vi "Main (DAQ, 3 Tasks, Event Messenger).vi"() -> ()   [LabVIEW 2018]
doc: "Datenerfassung - Producer/Consumer mit Zustandsmaschine und Tag Channel\n\n* Analoges Eingangssigna, Definition des\nDAQmx Kanals im NI Max\n* Realisierung mit eine Zustandsmaschine\n* Drei Schleifen (Tasks): Zustandsmaschine und Datenerfassung und Auswertung\n*Realisierung des User Interfaces mit Event Structure\n* Kommunikation benutzereingaben (Zustandsmaschine) zu Datenerfassung mit \"Tag Channel\" und \"Stream Channel\"\n* Anzeige der Events\n* Anzeige der Zustände \"Messung/Warten/Auswertung\""
uses:
  Type Definitions/States UI.ctl
  Type Definitions/MessungEvents.ctl
  <vilib>/DAQmx/read.llb/DAQmx Read (Analog Wfm 1Chan NSamp).vi
  <extravilib>/ChannelInstances/Stream-wfm(dbl)/Read With Abort.vi
  <extravilib>/ChannelInstances/Stream-wfm(dbl)/Write With Abort.vi
  <extravilib>/ChannelInstances/Stream-wfm(dbl)/EndpointRead.vi
  <extravilib>/ChannelInstances/Stream-wfm(dbl)/Endpoint.vi
  <extravilib>/ChannelInstances/Event Messenger-t'MessungEvents.ctl'/Instantiate.vi
  <extravilib>/ChannelInstances/Event Messenger-t'MessungEvents.ctl'/))Channel.vi
  <extravilib>/ChannelInstances/Stream-wfm(dbl)/Instantiate.vi
  <extravilib>/ChannelInstances/Stream-wfm(dbl)/)Channel.vi
  <resource>/ChannelSupport/_ChannelSupport/WaitIfNeeded.vi
  <vilib>/Waveform/WDTOps.llb/WDT Append Waveforms DBL.vi
  <vilib>/DAQmx/miscellaneous.llb/DAQmx Fill In Error Info.vi
  <extravilib>/ChannelInstances/Stream-wfm(dbl).lvlib
  <extravilib>/ChannelInstances/Event Messenger-t'MessungEvents.ctl'.lvlib
panel:
  in  "Tab Control":enum32{"Graph", "Chart"}(tab)=enum."Chart"
  out "element":waveform(dbl)(graph)
  out "Waveform Chart":waveform(dbl)(graph)
  out "Messung":bool
  out "Events":string="Exit= 1"
  in  "Messung":bool
  in  "Exit":bool
  out "Anzeige":dbl(knob) scale=0.0..10.0 scale format="%1.1f"
  # "Datenerfassung - Producer/Consumer mit Zustandsmaschine und Tag sowie Stream Channel\n\n* Analoges Eingangssignal, Definition des\nDAQmx Kanals im NI Max\n*  Realisierung mit eine Zustandsmaschine\n* Zustandsmaschine nur für UI Events\n* Drei Schleifen (Tasks): Zustandsmaschine, Datenerfassung und Auswertung\n*Realisierung des User Interfaces mit Event Structure\n* Kommunikation Benutzereingaben (Zustandsmaschine) zu Datenerfassung mit \"Event Messages\"\n* Daten per Stream Channel zum Zustand \"Auswertung\"\n* Anzeige der Events\n* Anzeige der Zustände \"Messung/Warten/Auswertung\"\n\nTiming\n* Task 1Khz Sampling Rate und 100 Samples\n* Gemessen jede 1sec (Timed loop)\n\nBug\nnur eine Scan!"
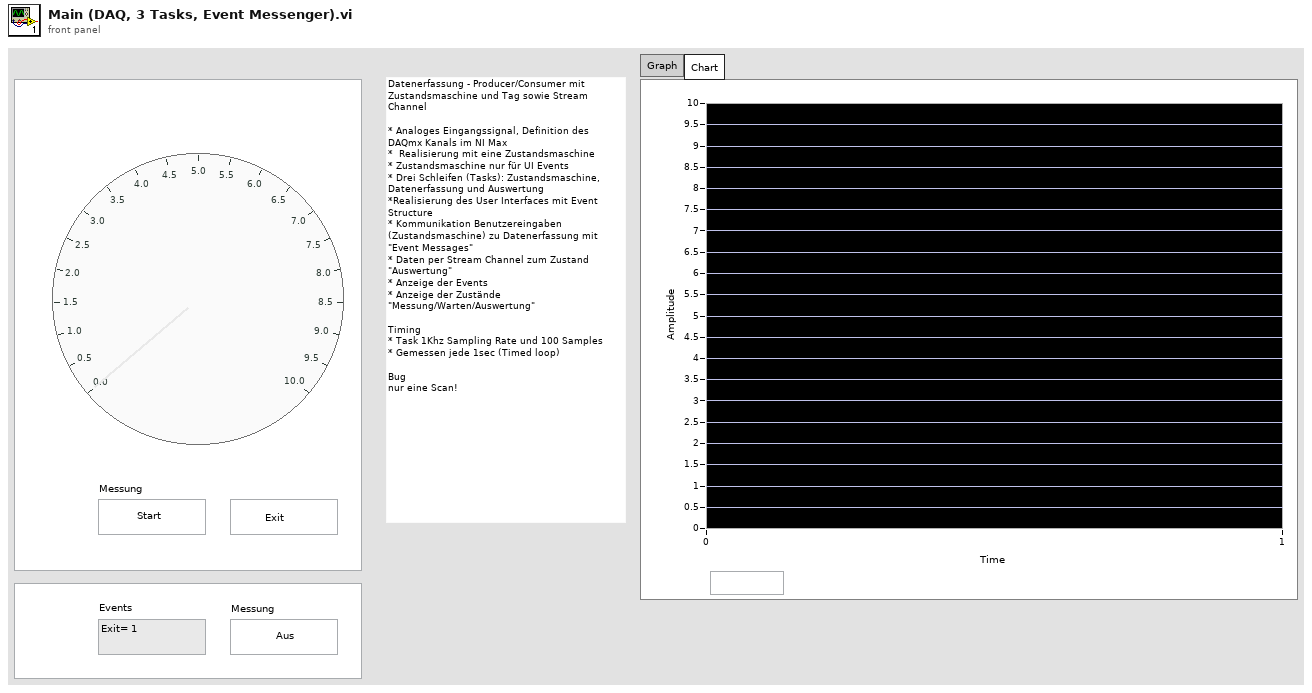
[diagram p1: front panel]
types:
  T1 = typedef "States UI.ctl" = enum16{"Initialize", "Wait for Event", "Exit"}
  T2 = typedef "MessungEvents.ctl" = enum16{"Starten", "Pausieren", "Stoppen"}
  T3 = typedef "Event Messenger-t'MessungEvents.ctl'.lvlib/))Channel.ctl" = refnum<queue>
  T4 = typedef "Stream-wfm(dbl).lvlib/)Channel.ctl" = refnum<queue>
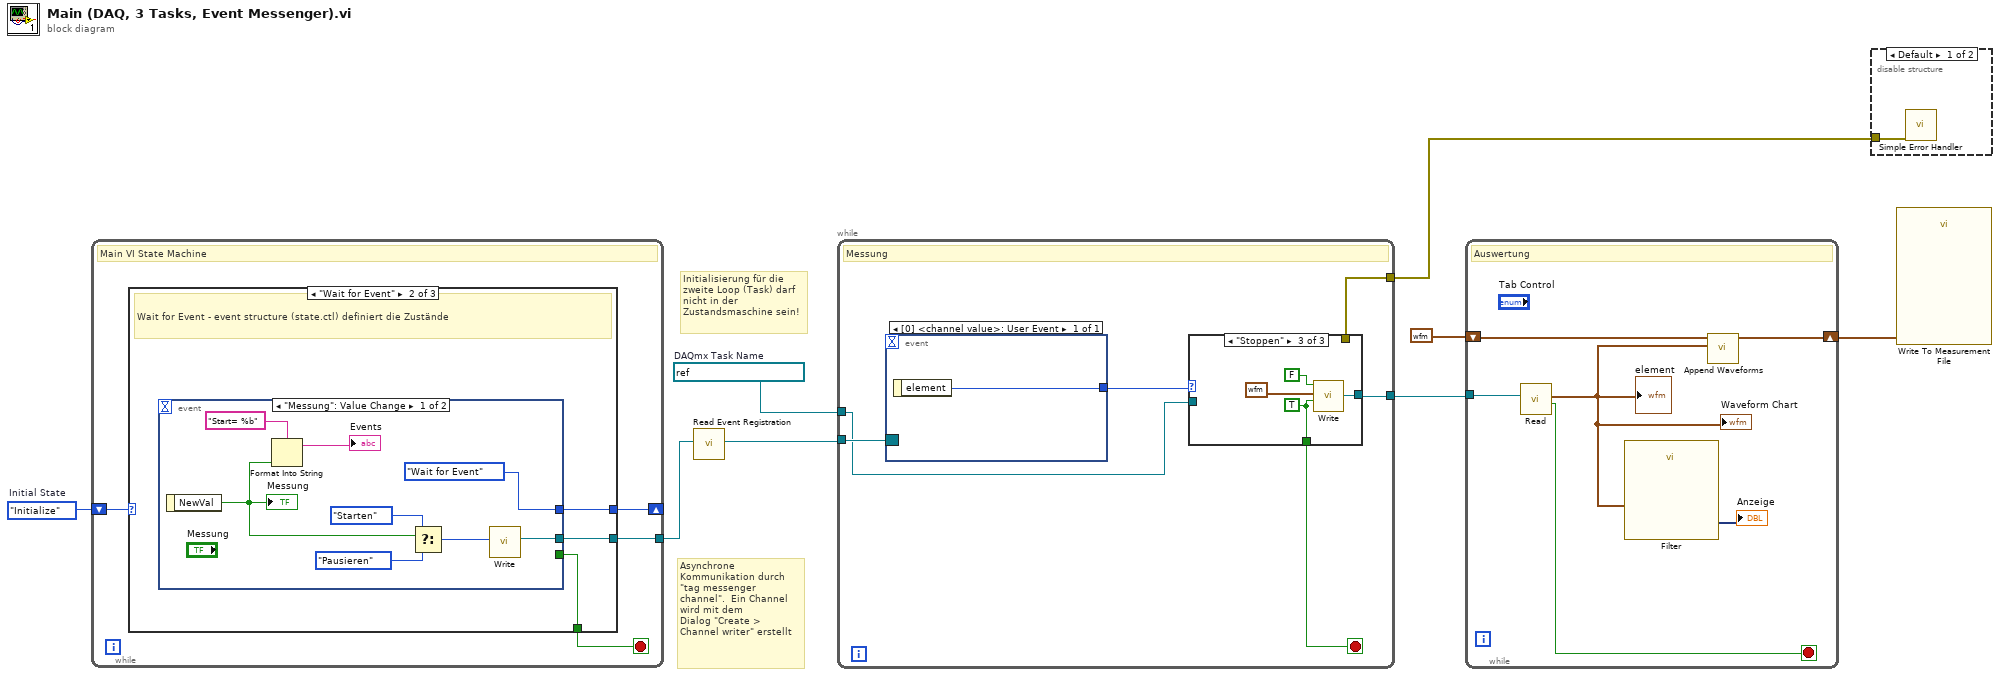
[diagram p0: block diagram]
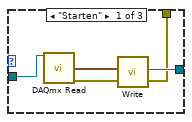
[diagram p2: hidden frame]
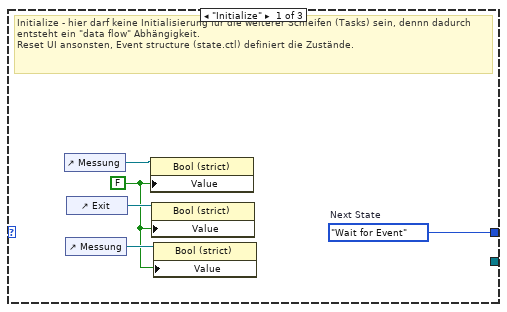
[diagram p4: hidden frame]
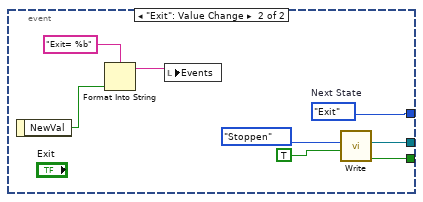
[diagram p5: hidden frame]
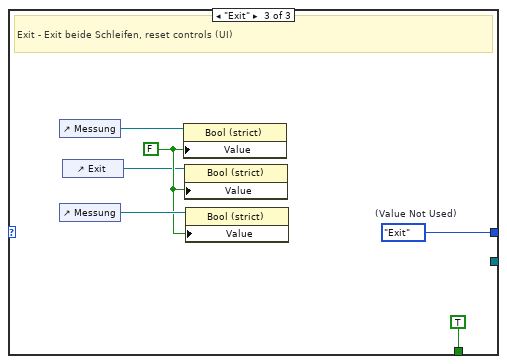
[diagram p6: hidden frame]
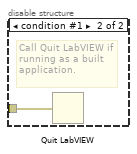
[diagram p7: hidden frame]
diagram:
  w6 = refnum<k21> "Spannung_1kHz100"  # DAQmx Task Name
  w8 = States_UI."Initialize"  # Initial State
  # "Initialisierung für die zweite Loop (Task) darf\nnicht in der Zustandsmaschine sein!"
  # "Asynchrone Kommunikation durch\n\"tag messenger channel\".  Ein Channel wird mit dem\nDialog \"Create > Channel writer\" erstellt"
  n1 = while {
    shift-right: [w11] -> _
    shift-left: w8 -> [w12]
    tunnel: [w9] -> w3
    stop <- w10 stop-if-true
    # "Main VI State Machine"
    n2 = case shown="\"Wait for Event\"" w12 {
      tunnel: [w17 w20 w42] -> w11
      tunnel: [_ w18 TRUE ("Stop Loop?")] -> w10
      tunnel: [_ w19 _] -> w9
      frame "Initialize" {
        w13 = FALSE ("Value")
        w17 = States_UI."Wait for Event"  # Next State
        # "Initialize - hier darf keine Initialisierung für die weiterer Schleifen (Tasks) sein, dennn dadurch entsteht ein \"data flow\" Abhängigkeit. \nReset UI ansonsten, Event structure (state.ctl) definiert die Zustände."
        n3 = control-ref of="Messung"() -> (w16:refnum<vi>)
        n4 = control-ref of="Messung"() -> (w14:refnum<vi>)
        n5 = control-ref of="Exit"() -> (w15:refnum<vi>)
        n6 = property class="Bool (strict)"(reference=w16, "Value"=w13) -> ()  [unwired: 1 in, 2 out]
        n7 = property class="Bool (strict)"(reference=w15, "Value"=w13) -> ()  [unwired: 1 in, 2 out]
        n8 = property class="Bool (strict)"(reference=w14, "Value"=w13) -> ()  [unwired: 1 in, 2 out]
      }
      frame "Wait for Event" {
        # "Wait for Event - event structure (state.ctl) definiert die Zustände"
        n9 = event shown="[0] \"Messung\": Value Change" {
          selector: _ -> [_ _]
          dyn-events: _ -> [_ _]
          timeout: _ -> [_ _]
          tunnel: [States_UI."Wait for Event" ("Next State") w36] -> w20
          tunnel: [w21 w32] -> w19
          tunnel: [_ w29] -> w18
          event "Messung": Value Change {
            n10 = event-data() -> ("NewVal"=w25:bool)  [unwired: 1 in]
            "Messung" <- w25
            n11 = Format Into String(format string="Start= %b", w25) -> (resulting string=→"Events":string)  [unwired: 2 in, 1 out]
            n12 = Select(t=MessungEvents."Starten" ("Messung Events"), s=w25, f=MessungEvents."Pausieren" ("Messung Events")) -> (s? t:f=w22:T2)
            n13 = call <extravilib>:"Write.vi"("element"=w22) -> ("channel"=w21:T3)  [unwired: 9 in, 1 out]
          }
          event "Exit": Value Change {
            w36 = States_UI."Exit"  # Next State
            n14 = event-data() -> ("NewVal"=w34:bool)  [unwired: 1 in]
            n15 = Format Into String(format string="Exit= %b", w34) -> (resulting string=w35:string)  [unwired: 2 in, 1 out]
            n16 = local write "Events"(w35) -> ()
            n17 = call <extravilib>:"Write.vi"("last element? (F)"=TRUE, "element"=MessungEvents."Stoppen" ("Messung Events")) -> ("done?"=w29:bool, "channel"=w32:T3)  [unwired: 8 in]
          }
        }
      }
      frame "Exit" {
        w39 = FALSE ("Value")
        w42 = States_UI."Exit"  # (Value Not Used)
        # "Exit - Exit beide Schleifen, reset controls (UI)"
        n18 = control-ref of="Messung"() -> (w41:refnum<vi>)
        n19 = control-ref of="Messung"() -> (w40:refnum<vi>)
        n20 = control-ref of="Exit"() -> (w38:refnum<vi>)
        n21 = property class="Bool (strict)"(reference=w41, "Value"=w39) -> ()  [unwired: 1 in, 2 out]
        n22 = property class="Bool (strict)"(reference=w38, "Value"=w39) -> ()  [unwired: 1 in, 2 out]
        n23 = property class="Bool (strict)"(reference=w40, "Value"=w39) -> ()  [unwired: 1 in, 2 out]
      }
    }
  }
  n24 = call <extravilib>:"Read Event Registration.vi"("channel"=w3) -> ("event registration refnum"=w2:refnum<event-registration>)  [unwired: 10 in]
  n25 = while {
    tunnel: [w46] -> w7
    tunnel: w6 -> [w45]
    tunnel: w2 -> [w48]
    tunnel: [w43] -> w1
    stop <- w44 stop-if-true
    # "Messung"
    n26 = event shown="[0] <channel value>: User Event" {
      selector: w48 -> [_]
      dyn-events: _ -> [_]
      timeout: _ -> [_]
      tunnel: [w57] -> w47
      event User Event {
        n27 = event-data() -> ("element"=w57:T2)  [unwired: 1 in]
      }
    }
    n28 = case shown="\"Stoppen\"" w47 {
      tunnel: [w51 _ w54] -> w46
      tunnel: w45 -> [w50 _ _]
      tunnel: [_ _ w53] -> w44
      tunnel: [w49 _ _] -> w43
      frame "Starten" {
        n29 = call-poly <vilib>:"DAQmx Read.vi"("task/channels in"=w50) -> ("data"=w52:waveform(dbl), "error out"=w49:errorcluster)  [unwired: 12 in, 1 out]
        n30 = call <extravilib>:"Write.vi"("element"=w52) -> ("channel"=w51:T4)  [unwired: 8 in, 2 out]
      }
      frame "Pausieren" {
      }
      frame "Stoppen" {
        w53 = TRUE ("abort")
        n31 = call <extravilib>:"Write.vi"("last element? (F)"=w53, "element"=waveform(dbl) {"t0"=timestamp(0 s since 1904-01-01), "dt"=1.0, "Y"=[]}, "element valid? (T)"=FALSE) -> ("channel"=w54:T4)  [unwired: 6 in, 2 out]
      }
    }
  }
  n32 = while {
    tunnel: w7 -> [w63]
    shift-right: [w60] -> w4
    shift-left: waveform(dbl) {"t0"=timestamp(0 s since 1904-01-01), "dt"=1.0, "Y"=[]} ("Waveform") -> [w61]
    stop <- w58 stop-if-true
    # "Auswertung"
    n33 = call <extravilib>:"Read.vi"("channel"=w63) -> ("last element?"=w58:bool, "element"=w62:waveform(dbl))  [unwired: 6 in, 3 out]
    "element" <- w62
    "Waveform Chart" <- w62
    n34 = call "Filter"("Signal"=w62) -> ("Filtered Signal"=→"Anzeige":dynamicdata)  [unwired: 9 in, 1 out]
    n35 = call-poly <vilib>:"Append Waveforms.vi"("waveform B"=w62, "waveform A"=w61) -> ("waveform out"=w60:waveform(dbl))  [unwired: 8 in, 1 out]
  }
  n36 = disable-structure shown="Default" {
    disable-tunnel: w1 -> [w64 w65]
    frame condition #0 (active) {
      n37 = call <vilib>:"Simple Error Handler.vi"("error in (no error)"=w64) -> ()  [unwired: 4 in, 5 out]
    }
    frame condition #1 {
      # "Call Quit LabVIEW if running as a built application."
      n38 = Quit LabVIEW(quit? (T)=w65) -> ()
    }
  }
  n39 = call "Write To Measurement File"("Signals"=w4) -> ()  [unwired: 16 in, 3 out]
